vi "Get Result.vi"(6 "Last request":bool, 8 "error in (no error)":errorcluster, 11 "Instrument Recorder in":refnum<class "Ruby Spectra.lvclass">) -> (0 "error out":errorcluster, 2 "Result":refnum<class "Acquired Result.lvclass">, 3 "Instrument Recorder out":refnum<class "Ruby Spectra.lvclass">)   [LabVIEW 2018, in "Ruby Spectra.lvclass"]
uses:
  Ruby Spectra.lvclass
  C:/github/2018/LabActor/Recorders/Spectrometer/Spectrometer.lvclass
  NHMFL_Core/Libraries/Instruments/Results/Acquired Result/Acquired Result.lvclass
  Spectrometer/Spectrometer.lvclass/Spectrometer.ctl
  NHMFL_Core/Libraries/Instruments/Spectrometer Driver/Spectrometer Driver.lvclass/Spectrometer Driver.ctl
  Spectrometer/Read Spectrum Graph ref.vi
  NHMFL_Core/Libraries/Instruments/Spectrometer Driver/Read Spectrum plot.vi
  Spectrometer/Read Spectrometer Driver.lvclass.vi
  Spectrometer/Spectrometer.lvclass
  NHMFL_Core/Libraries/Instruments/Spectrometer Driver/Spectrometer Driver.lvclass
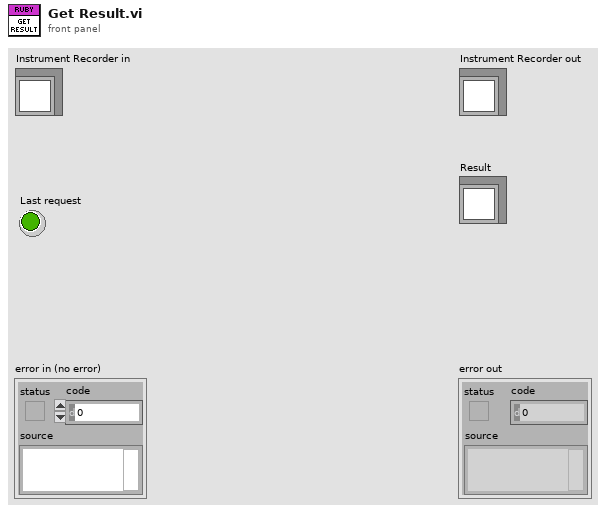
[diagram p1: front panel]
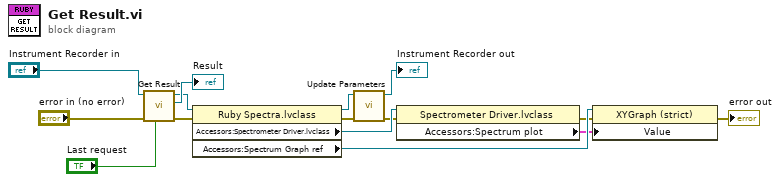
[diagram p0: block diagram]
diagram:
  n1 = call-parent "Get Result.vi"("Last request"="Last request", "error in (no error)"="error in (no error)", "Instrument Recorder in"="Instrument Recorder in") -> ("error out"=w6:errorcluster, "Result"=→"Result":refnum<class "Acquired Result.lvclass">, "Instrument Recorder out"=w7:refnum<class "Ruby Spectra.lvclass">)  [unwired: 6 in]
  n2 = property class="Ruby Spectra.lvclass"(reference=w7, error in=w6) -> (reference out=w4:refnum<class "Ruby Spectra.lvclass">, error out=w2:errorcluster, "Accessors:Spectrometer Driver.lvclass"=w11:refnum<class "Spectrometer Driver.lvclass">, "Accessors:Spectrum Graph ref"=w10:refnum<vi>)
  n3 = call-dynamic "Update Parameters.vi"("error in (no error)"=w2, "Ruby Spectra in"=w4) -> ("error out"=w1:errorcluster, "Ruby Spectra out"=→"Instrument Recorder out":refnum<class "Ruby Spectra.lvclass">)  [unwired: 8 in]
  n4 = property class="Spectrometer Driver.lvclass"(reference=w11, error in=w1) -> (error out=w8:errorcluster, "Accessors:Spectrum plot"=w9:cluster{"Array":dbl[], "Array":dbl[]}[])  [unwired: 1 out]
  n5 = property class="XYGraph (strict)"(reference=w10, error in=w8, "Value"=w9) -> (error out=→"error out":errorcluster)  [unwired: 1 out]
